vi "ArmUp.vi"() -> ()   [LabVIEW 2018]
panel:
  in  "ArmRaise":bool
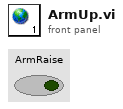
[diagram p1: front panel]
diagram:
